vi "fastseq_slot_to_orders.vi"(1 "Add empty slots":bool, 2 "Fast sequence":dbl[][](array[numeric])) -> (0 "Orders":u64[](array[numeric]))   [LabVIEW 2013]
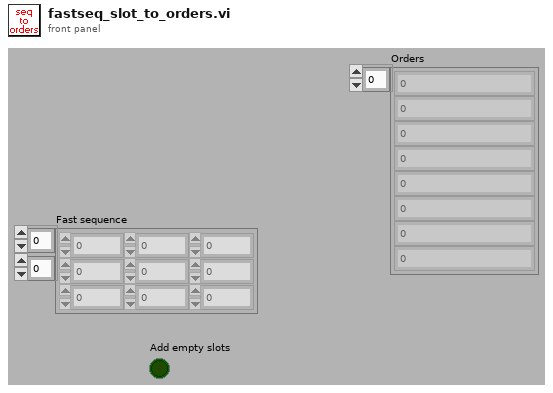
[diagram p1: front panel]
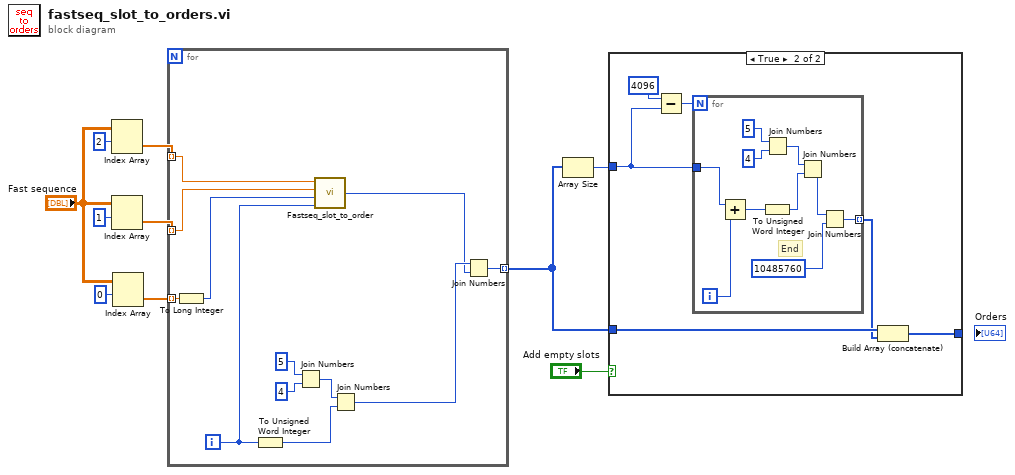
[diagram p0: block diagram]
diagram:
  n1 = Index Array(array="Fast sequence", index (row)=2) -> (element=w4:dbl[])  [unwired: 1 in]
  n2 = Index Array(array="Fast sequence", index (row)=1) -> (element=w5:dbl[])  [unwired: 1 in]
  n3 = Index Array(array="Fast sequence", index (row)=0) -> (element=w6:dbl[])  [unwired: 1 in]
  n4 = for {
    tunnel: w6 -> [w22] mode=indexing
    tunnel: w5 -> [w21] mode=indexing
    tunnel: w4 -> [w20] mode=indexing
    tunnel: [w13] -> w2 mode=indexing
    i -> [w11]
    n5 = To Long Integer(number=w22) -> (32bit integer=w19:i32)
    n6 = To Unsigned Word Integer(number=w11) -> (unsigned 16bit integer=w15:u16)
    n7 = Join Numbers(hi=u8 5, lo=u8 4) -> ((hi.lo)=w16:u16)
    n8 = call "Fastseq_slot_to_order.vi"("index"=w11, "Type"=w19, "data1"=w21, "data2"=w20) -> ("Order"=w12:u64)
    n9 = Join Numbers(hi=w16, lo=w15) -> ((hi.lo)=w14:u32)
    n10 = Join Numbers(hi=w14, lo=w12) -> ((hi.lo)=w13:u64)
  }
  n11 = Array Size(array=w2) -> (size(s)=w1:i32)
  n12 = case shown="True" "Add empty slots" {
    tunnel: w2 -> [w23 w29]
    tunnel: [w23 w25] -> _
    tunnel: w1 -> [_ w26]
    frame False {
    }
    frame True {
      n13 = Subtract(x=4096, y=w26) -> (x-y=w27:i32)
      n14 = for {
        N: w27 -> [_]
        tunnel: w26 -> [w34]
        tunnel: [w30] -> w24 mode=indexing
        i -> [w35]
        # "End"
        n15 = Add(x=w34, y=w35) -> (x+y=w33:i32)
        n16 = To Unsigned Word Integer(number=w33) -> (unsigned 16bit integer=w39:u16)
        n17 = Join Numbers(hi=u8 5, lo=u8 4) -> ((hi.lo)=w38:u16)
        n18 = Join Numbers(hi=w38, lo=w39) -> ((hi.lo)=w32:u32)
        n19 = Join Numbers(hi=w32, lo=u32 10485760) -> ((hi.lo)=w30:u64)
      }
      n20 = Build Array (concatenate)(w29, w24) -> (w25:u64[])
    }
  }
